vi "FakeBeamProfileGenerator.vi"(5 "w_0":dbl=0.002, 7 "Z_0":dbl=0.1, 9 "Z":dbl=1.0, 10 "Y":dbl) -> (2 "E":dbl)   [LabVIEW 2013]
doc: "This template is the starting point for creating a model function to be passed to the Nonlinear Curve Fit.vi."
uses:
  <vilib>/gmath/NI_Gmath.lvlib
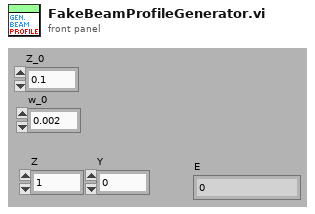
[diagram p1: front panel]
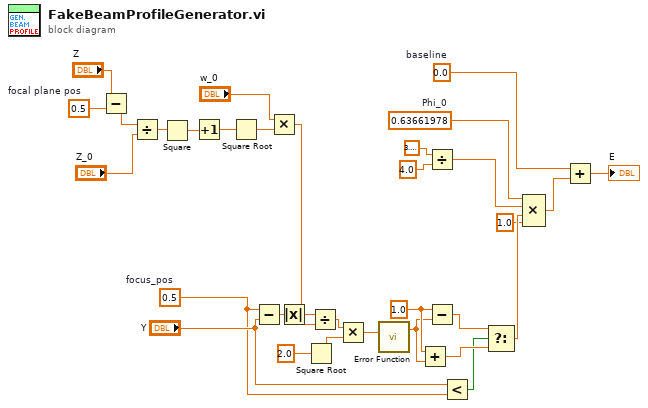
[diagram p0: block diagram]
diagram:
  w2 = 0.5  # focal plane pos
  w13 = 0.5  # focus_pos
  w7 = 0.0  # baseline
  w8 = 0.63661978  # Phi_0
  w20 = 1.0 ("x")
  n1 = Subtract(x="Z", y=w2) -> (x-y=w3:dbl)
  n2 = Divide(x=w3, y="Z_0") -> (x/y=w27:dbl)
  n3 = Square(x=w27) -> (x^2=w4:dbl)
  n4 = Increment(x=w4) -> (x+1=w26:dbl)
  n5 = Square Root(x=w26) -> (sqrt(x)=w12:dbl)
  n6 = Subtract(x=w13, y="Y") -> (x-y=w24:dbl)
  n7 = Multiply(x="w_0", y=w12) -> (x*y=w10:dbl)
  n8 = Absolute Value(x=w24) -> (abs(x)=w23:dbl)
  n9 = Square Root(x=2.0) -> (sqrt(x)=w31:dbl)
  n10 = Divide(x=w23, y=w10) -> (x/y=w22:dbl)
  n11 = Multiply(x=w22, y=w31) -> (x*y=w21:dbl)
  n12 = call <vilib>:"Error Function.vi"("x"=w21) -> ("erf(x)"=w19:dbl)  [unwired: 2 in]
  n13 = Add(x=w20, y=w19) -> (x+y=w17:dbl)
  n14 = Divide(x=3.141592653589793, y=4.0) -> (x/y=w28:dbl)
  n15 = Subtract(x=w20, y=w19) -> (x-y=w18:dbl)
  n16 = Less?(x="Y", y=w13) -> (x < y?=w16:bool)
  n17 = Select(t=w18, s=w16, f=w17) -> (s? t:f=w15:dbl)
  n18 = Compound Arithmetic op=MULTIPLY(w8, w28, w15, 1.0 ("value")) -> (w25:dbl)
  n19 = Add(x=w7, y=w25) -> (x+y=→"E":dbl)
